vi "Instantiate Py Shell.vi"(11 "error in (no error)":errorcluster) -> (4 "Document.lvclass":refnum<class "Document.lvclass">, 15 "error out":errorcluster)   [LabVIEW 2016, in "Py Shell.lvclass"]
uses:
  Py Shell.lvclass
  Document.lvclass
  D:/MDI Project/source code/Document/Document.lvclass
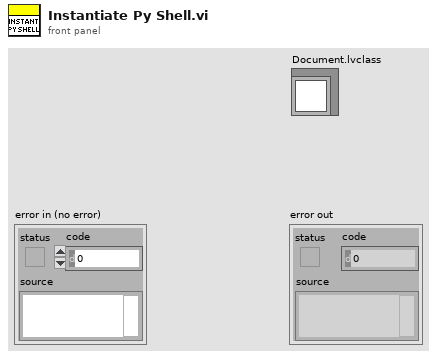
[diagram p1: front panel]
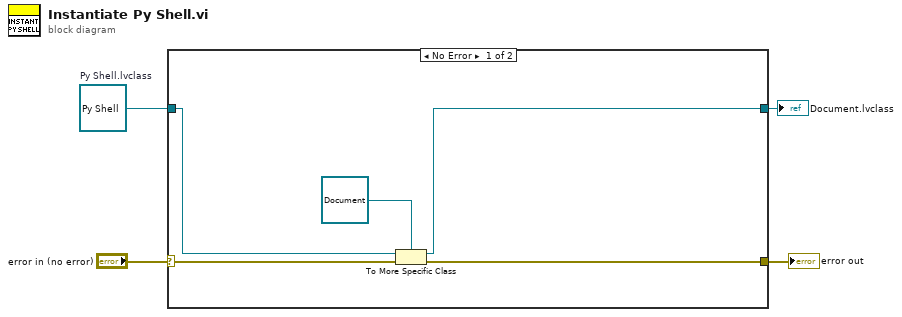
[diagram p0: block diagram]
diagram:
  w2 = refnum<class "Py Shell.lvclass"> refnum  # Py Shell.lvclass
  n1 = case shown="No Error" "error in (no error)" {
    selector: "error in (no error)" -> [w9 w11]
    tunnel: [w8 w11] -> w3
    tunnel: [w7 w10] -> w1
    tunnel: w2 -> [w5 w10]
    frame No Error {
      n2 = To More Specific Class(target class=refnum<class "Document.lvclass"> refnum ("Document.lvclass"), reference=w5, error in=w9) -> (specific class reference=w7:refnum<class "Document.lvclass">, error out=w8:errorcluster)
    }
    frame Error {
    }
  }
  "error out" <- w3
  "Document.lvclass" <- w1
